vi "DB Insert.vi"(6 "Schema Name":string, 7 "Data":string[][](array[string]), 8 "error in (no error)":errorcluster, 9 "columns":string[](array[string]), 10 "table":string, 11 "Database in":refnum<class "Database.lvclass">) -> (0 "error out":errorcluster, 2 "SQL":string caption="SQL+ (Col[]) VALUES (?[])", 3 "Database out":refnum<class "Database.lvclass">)   [LabVIEW 2023, in "HardwareAbstractionLayer_LVOOP.lvlib" / "Database.lvclass"]
doc: "This VI is DB SQL Insert Query"
uses:
  Database.lvclass
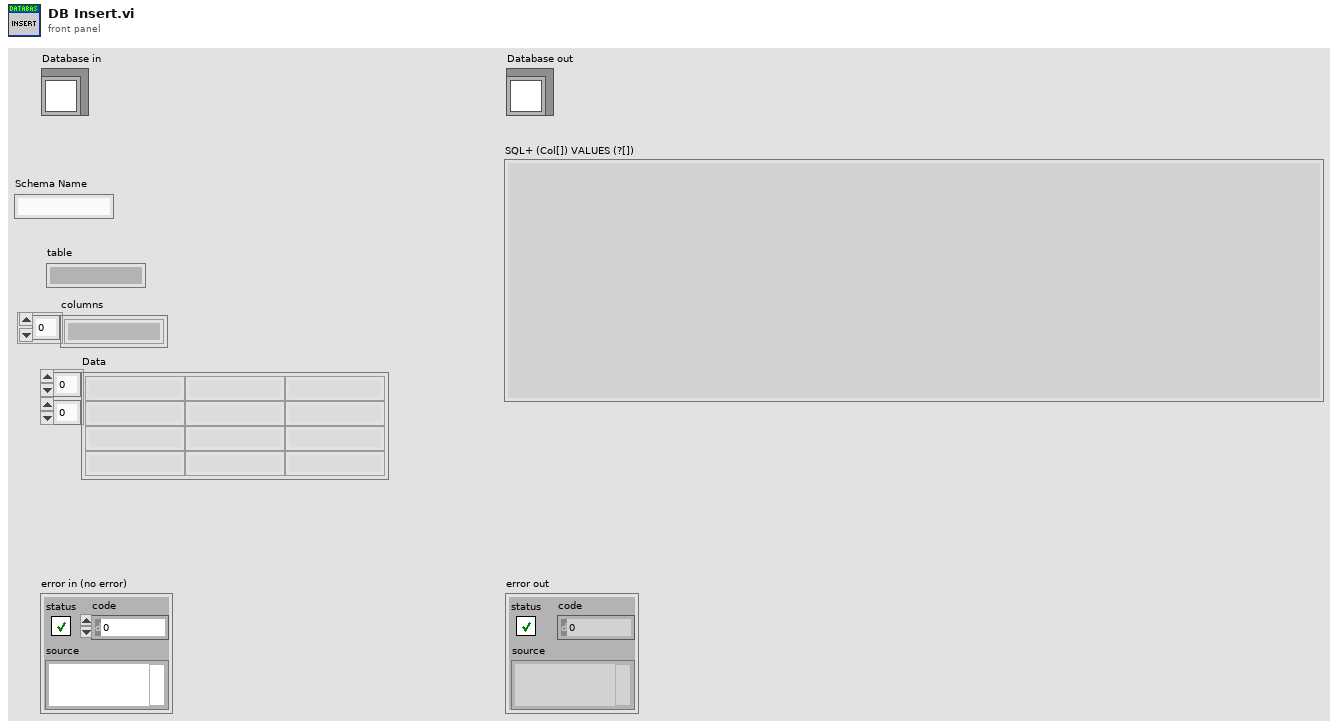
[diagram p1: front panel]
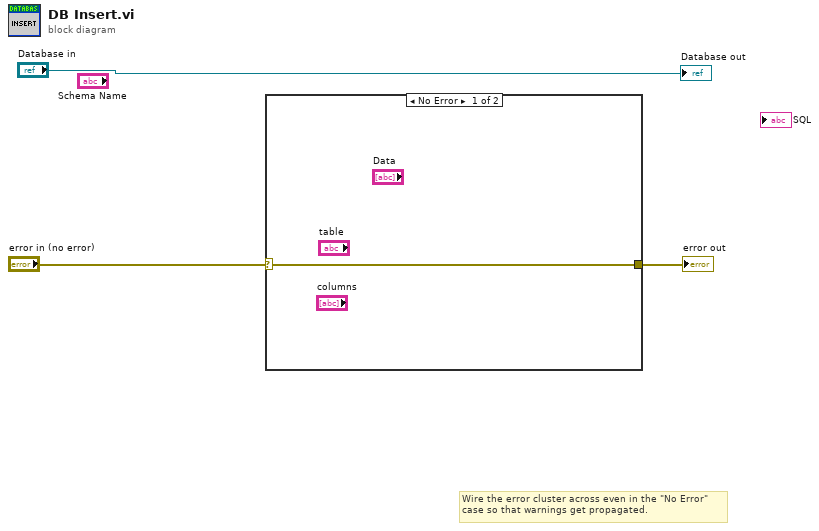
[diagram p0: block diagram]
diagram:
  # "Wire the error cluster across even in the \"No Error\"\ncase so that warnings get propagated."
  n1 = case shown="No Error" "error in (no error)" {
    selector: "error in (no error)" -> [w4 w5]
    tunnel: [w4 w5] -> w1
    frame No Error {
    }
    frame Error {
    }
  }
  "error out" <- w1
  "Database out" <- "Database in"
